vi "Reset stages speed.vi"(8 "error in (no error)":errorcluster, 11 "Tomo in":refnum<class "Tomo.lvclass">) -> (0 "error out":errorcluster, 3 "Tomo out":refnum<class "Tomo.lvclass">)   [LabVIEW 2012, in "Tomo.lvclass"]
uses:
  Tomo.lvclass
  <vilib>/Distrio/Murmex/Murmex/Murmex.lvclass
  <vilib>/Distrio/Murmex/Murmex/update_cluster.ctl
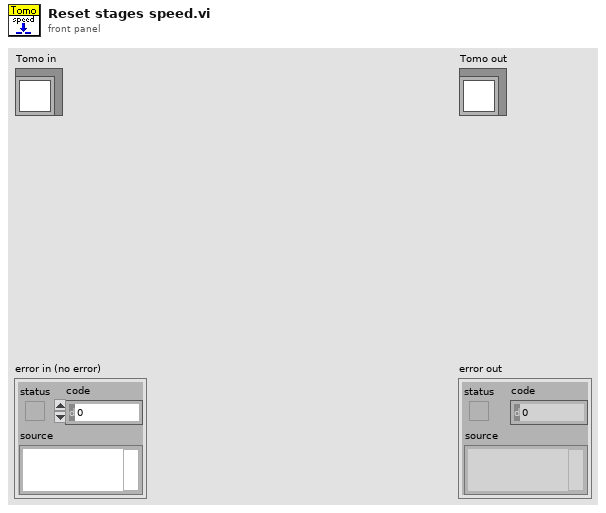
[diagram p1: front panel]
types:
  T1 = typedef "Murmex.lvlib/Murmex.lvclass/update_cluster.ctl" = cluster{"target ID":string, "key chains":string[], "values":variant[]}
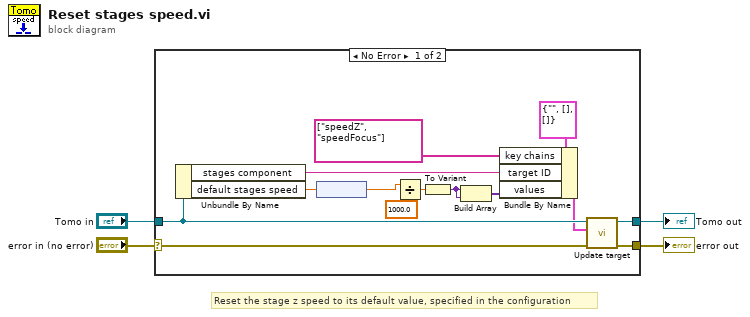
[diagram p0: block diagram]
diagram:
  # "Reset the stage z speed to its default value, specified in the configuration"
  n1 = case shown="No Error" "error in (no error)" {
    selector: "error in (no error)" -> [w17 w20]
    tunnel: [w16 w20] -> w3
    tunnel: [w14 w19] -> w1
    tunnel: "Tomo in" -> [w15 w19]
    frame No Error {
      n2 = Unbundle By Name(w15) -> ("stages component"=w11:string, "default stages speed"=w13:dbl[unit])
      n3 = node(w13) -> (w7:dbl)
      n4 = Divide(x=w7, y=1000.0) -> (x/y=w6:dbl)
      n5 = To Variant(anything=w6) -> (Variant=w5:variant)
      n6 = Build Array(w5, w5) -> (w12:variant[])
      n7 = Bundle By Name(cluster=T1 {"target ID"="", "key chains"=[], "values"=[]} ("update cluster"), "key chains"=string[] ["speedZ", "speedFocus"], "target ID"=w11, "values"=w12) -> (w9:T1)
      n8 = call <vilib>:"Update target.vi"("error in (no error)"=w17, "update cluster"=w9, "MurmexBase in"=w15) -> ("error out"=w16:errorcluster, "MurmexBase out"=w14:refnum<class "Tomo.lvclass">)  [unwired: 7 in]
    }
    frame Error {
    }
  }
  "error out" <- w3
  "Tomo out" <- w1
